vi "06MAR.vi"(0 "File Path":path) -> (1 "lowercase file extension":string, 2 "new picture":picture, 3 "new picture 2":picture)   [LabVIEW 2020]
doc: "SubVI para adquirir imagen"
panel:
  out "Array":u8[][](array[numeric])
  in  "Enum":T1(ring)
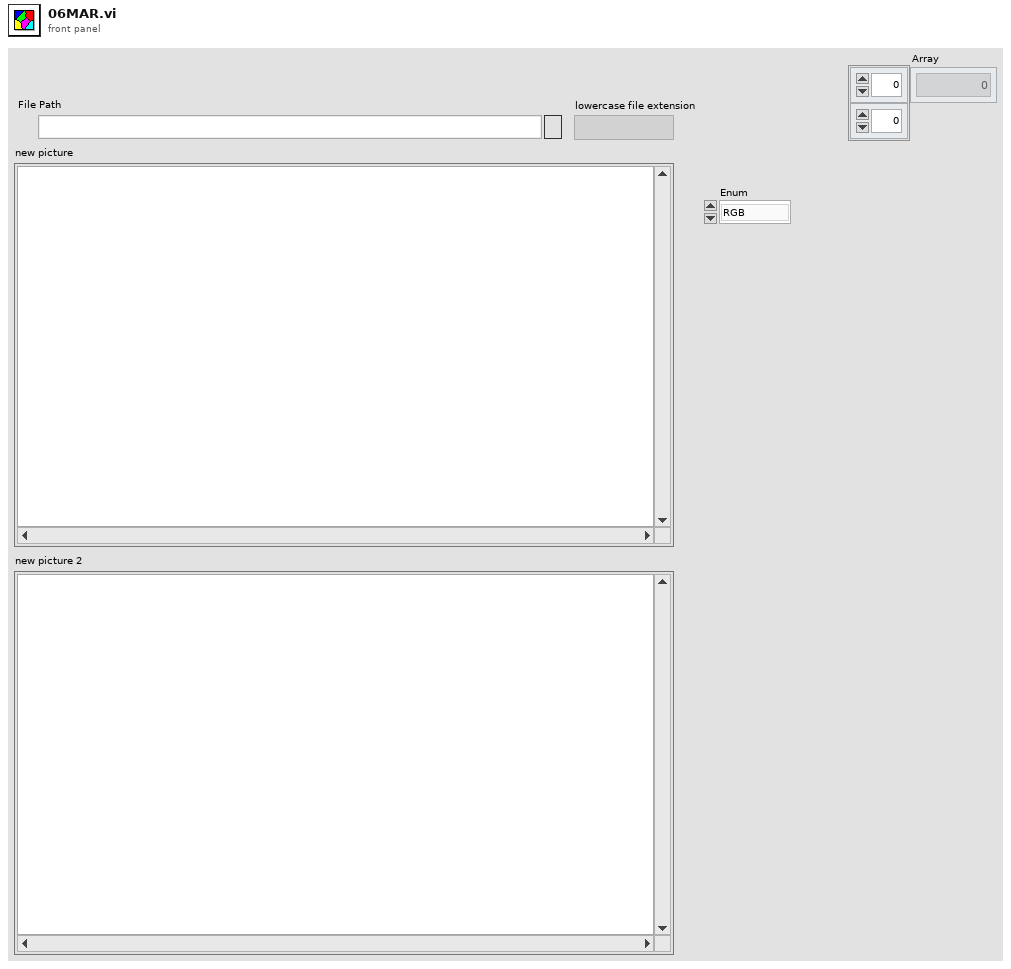
[diagram p1: front panel]
types:
  T1 = enum16{"RGB", "R", "G", "B", "C", "M", "Y", "H", "S", "V", "I", "YI", "II", "Q", ""}
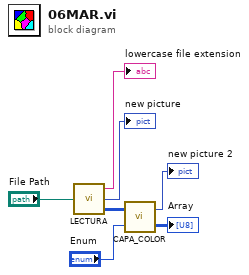
[diagram p0: block diagram]
diagram:
  n1 = call "LECTURA.vi"("File Path"="File Path") -> ("lowercase file extension"=→"lowercase file extension":string, "new picture"=→"new picture":picture, "24-bit pixmap"=w4:u32[][])
  n2 = call <userlib>:"CAPA_COLOR.vi"("Enum"="Enum", "24-bit pixmap"=w4) -> ("Array"=→"Array":u8[][], "new picture"=→"new picture 2":picture)
